vi "Destroy.vi"(8 "error in":errorcluster, 11 "Potting Procedure in":refnum<class "Potting Procedure.lvclass">) -> (0 "error out":errorcluster)   [LabVIEW 2011, in "Potting Procedure.lvclass"]
uses:
  Potting Procedure.lvclass
  Potting Procedure.lvclass/Potting Procedure.ctl
  Shared Components/Gantry Class/Gantry Class.lvclass
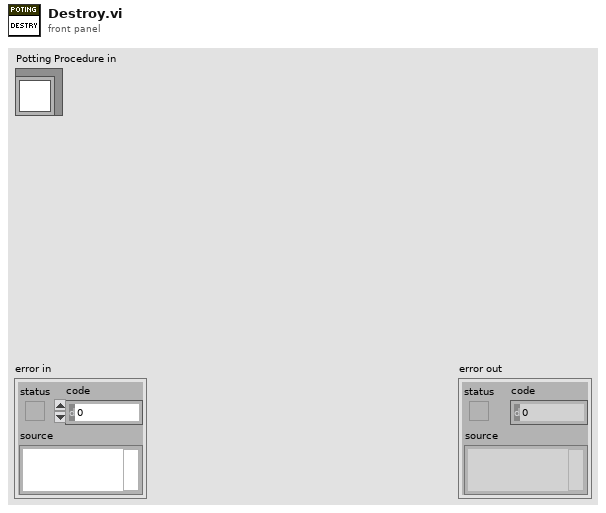
[diagram p1: front panel]
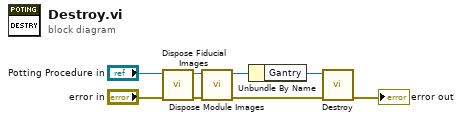
[diagram p0: block diagram]
diagram:
  n1 = call-dynamic "Dispose Fiducial Images.vi"("error in"="error in", "Potting Procedure in"="Potting Procedure in") -> ("error out"=w6:errorcluster, "Potting Procedure out"=w5:refnum<class "Potting Procedure.lvclass">)  [unwired: 8 in]
  n2 = call-dynamic "Dispose Module Images.vi"("error in"=w6, "Potting Procedure in"=w5) -> ("error out"=w1:errorcluster, "Potting Procedure out"=w3:refnum<class "Potting Procedure.lvclass">)  [unwired: 8 in]
  n3 = Unbundle By Name(w3) -> ("Gantry"=w8:refnum<class "Gantry Class.lvclass">)
  n4 = call "Destroy.vi"("error in"=w1, "Gantry Class in"=w8) -> ("error out"=→"error out":errorcluster)  [unwired: 9 in]
